vi "oa_TV Set Channel Info (Waveform Output NChan).vi"(4 "dt":dbl[](array[numeric]), 6 "t0":dbl[](array[numeric]), 7 "torisional vibration unit (RPM)":enum16{"RPM", "deg/s", "rad/s"}(ring), 8 "error in (no error)":errorcluster, 9 "pulse position":cluster{dbl[]}[](array[cluster]), 10 "seconds/revolution":cluster{dbl[]}[](array[cluster]), 11 "revolutions/minute":cluster{dbl[]}[](array[cluster])) -> (0 "error out":errorcluster, 1 "unit labels":string[](array[string]), 2 "speed profile":T1[](array[typedef]) {"speed [RPM]" format="%.2f"; "time [s]" format="%.2f"}, 3 "torsional vibration":waveform(dbl)[](array[waveform]))   [LabVIEW 2017, in "SoundVib_Torsional.lvlib"]
uses:
  <vilib>/addons/Sound and Vibration/Order Analysis/Torsional Vibration/SoundVib_Torsional.lvlib
  <vilib>/addons/Sound and Vibration/Order Analysis/Tach Process/SubVIs/speed profile.ctl
  <vilib>/addons/Sound and Vibration/Order Analysis/Tach Process/SoundVib_TachProcess.lvlib
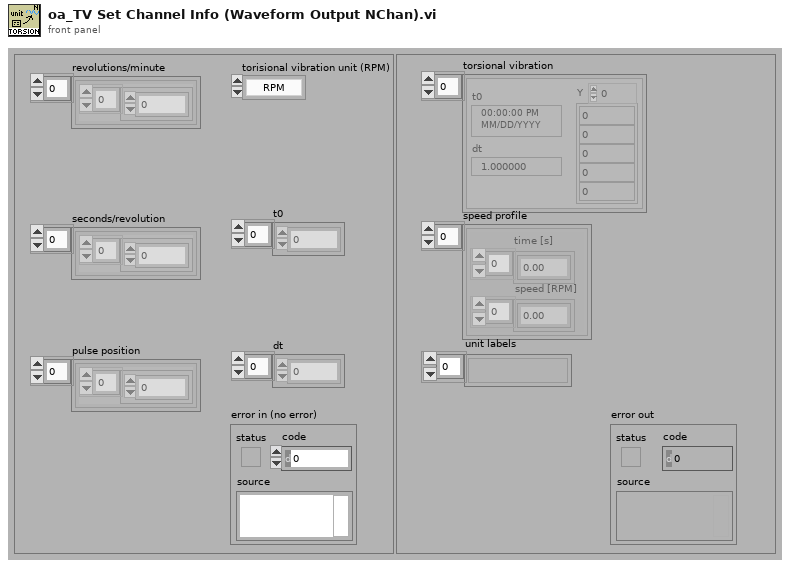
[diagram p1: front panel]
types:
  T1 = typedef "SoundVib_TachProcess.lvlib/speed profile.ctl" = cluster{"time [s]":dbl[], "speed [RPM]":dbl[]}
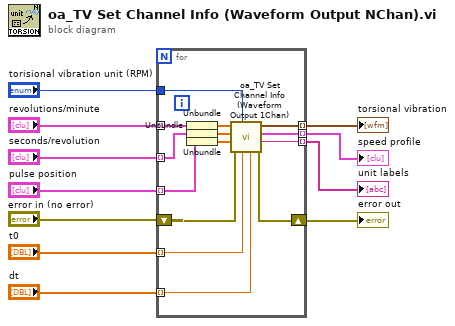
[diagram p0: block diagram]
diagram:
  n1 = for {
    shift-right: [w20] -> w10
    shift-left: "error in (no error)" -> [w21]
    tunnel: "revolutions/minute" -> [w25] mode=indexing
    tunnel: "t0" -> [w17] mode=indexing
    tunnel: "dt" -> [w16] mode=indexing
    tunnel: "seconds/revolution" -> [w22] mode=indexing
    tunnel: "torisional vibration unit (RPM)" -> [w15]
    tunnel: [w19] -> w5 mode=indexing
    tunnel: [w18] -> w4 mode=indexing
    tunnel: "pulse position" -> [w14] mode=indexing
    tunnel: [w12] -> w1 mode=indexing
    n2 = Unbundle(w25) -> (w24:dbl[])
    n3 = Unbundle(w22) -> (w23:dbl[])
    n4 = Unbundle(w14) -> (w13:dbl[])
    n5 = call <vilib>:"oa_TV Set Channel Info (Waveform Output 1Chan).vi"("output interval [s]"=w16, "t0"=w17, "torisional vibration unit (RPM)"=w15, "error in (no error)"=w21, "pulse position"=w13, "seconds/rev"=w23, "revolutions/sec"=w24) -> ("error out"=w20:errorcluster, "unit label"=w12:string, "speed profile"=w18:T1, "torsional vibration"=w19:waveform(dbl))  [unwired: 1 in]
  }
  "torsional vibration" <- w5
  "error out" <- w10
  "speed profile" <- w4
  "unit labels" <- w1
